vi "Clear Folder.vi"(8 "error in (no error)":errorcluster, 10 "Skip List":string[](array[string]), 11 "Path":path) -> (0 "error out":errorcluster)   [LabVIEW 2012]
doc: "SciScan 1.2 160622\nThis VI clears all the files in a specified folder; Except those specified in the 'Skip List'"
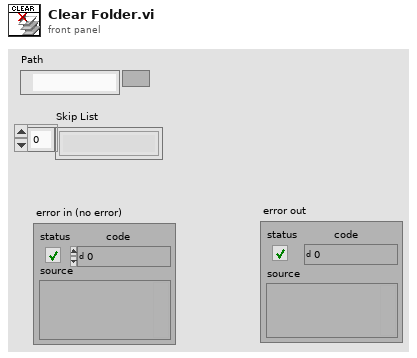
[diagram p1: front panel]
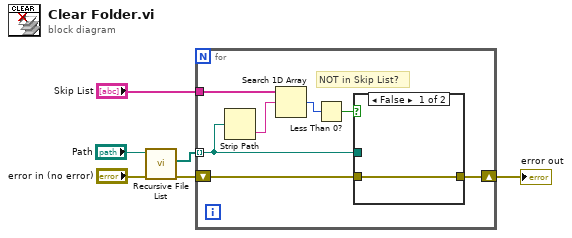
[diagram p0: block diagram]
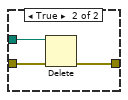
[diagram p2: hidden frame]
diagram:
  n1 = call <vilib>:"Recursive File List.vi"("error in (no error)"="error in (no error)", "Folder Path"="Path") -> ("error out"=w5:errorcluster, "All Files in Dir"=w6:path[])  [unwired: 5 in, 3 out]
  n2 = for {
    shift-right: [w13] -> w1
    shift-left: w5 -> [w12]
    tunnel: w6 -> [w11] mode=indexing
    tunnel: "Skip List" -> [w10]
    # "NOT in Skip List?"
    n3 = Strip Path(path=w11) -> (name=w9:string)  [unwired: 1 out]
    n4 = Search 1D Array(1D array=w10, element=w9) -> (index of element=w8:i32)  [unwired: 1 in]
    n5 = Less Than 0?(x=w8) -> (x < 0?=w7:bool)
    n6 = case shown="False" w7 {
      tunnel: [w14 w17] -> w13
      tunnel: w12 -> [w14 w16]
      tunnel: w11 -> [_ w15]
      frame False {
      }
      frame True {
        n7 = Delete(path (use dialog)=w15, error in=w16) -> (error out=w17:errorcluster)  [unwired: 3 in, 2 out]
      }
    }
  }
  "error out" <- w1
